vi "Check Lamp Status.vi"(8 "error in (no error)":errorcluster {"code" format="%.0x"}, 10 "Device Number (1)":i32=1, 11 "VISA Resource Name":refnum<visa-resource-name>) -> (0 "error out":errorcluster {"code" format="%.0x"}, 2 "Lamp Status":bool=TRUE, 3 "VISA Resource Name Out":refnum<visa-resource-name>)   [LabVIEW 2018, in "Olympus IX BX Series.lvlib"]
doc: "Gets the lamp status."
uses:
  Olympus IX BX Series.lvlib
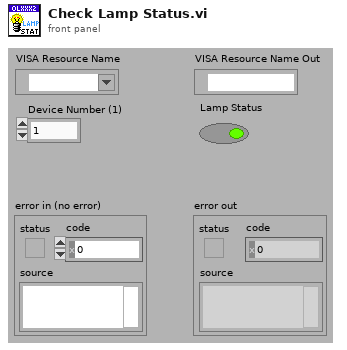
[diagram p1: front panel]
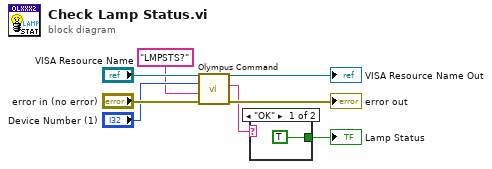
[diagram p0: block diagram]
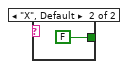
[diagram p2: hidden frame]
diagram:
  n1 = call "Olympus Command.vi"("error in (no error)"="error in (no error)", "Command string"="LMPSTS?" ("format string"), "Device Number (1)"="Device Number (1)", "VISA Resource Name"="VISA Resource Name") -> ("error out"=→"error out":errorcluster, "Result"=w1:string, "VISA Resource Name Out"=→"VISA Resource Name Out":refnum<visa-resource-name>)  [unwired: 5 in]
  n2 = case shown="\"OK\"" w1 {
    tunnel: [TRUE FALSE] -> w2
    frame "OK" {
    }
    frame "X", Default {
    }
  }
  "Lamp Status" <- w2
